vi "Modbus RT Driver DEBUG Simulate Data.vi"(8 "error in (no error)":errorcluster) -> (0 "error out":errorcluster, 1 "DEBUG RT-FIFOs Indexes":T2[](array[typedef]), 2 "DEBUG Modbus Items":T4[](array[typedef]), 5 "Input Specified Channel Ref List":T1[](array[typedef]) format="%.0x", 7 "Output Specified Channel Ref List":T1[](array[typedef]) format="%.0x")   [LabVIEW 2014, in "Modbus Engine.lvlib"]
uses:
  Modbus Engine.lvlib
  XML Deserializer/XML VIs/API/Controls/Modbus_Items.ctl
  XML Deserializer/XML VIs/API/Controls/Modbus_Item_Type.ctl
  Shared/FIFO Indexes.ctl
  <vilib>/NI Veristand/Custom Device API/Custom Device Channel Type.ctl
  <vilib>/NI Veristand/Custom Device API/Custom Device Item Ref.ctl
  <vilib>/NI Veristand/Custom Device API/Custom Device API.lvlib
  Shared/Modbus Shared.lvlib
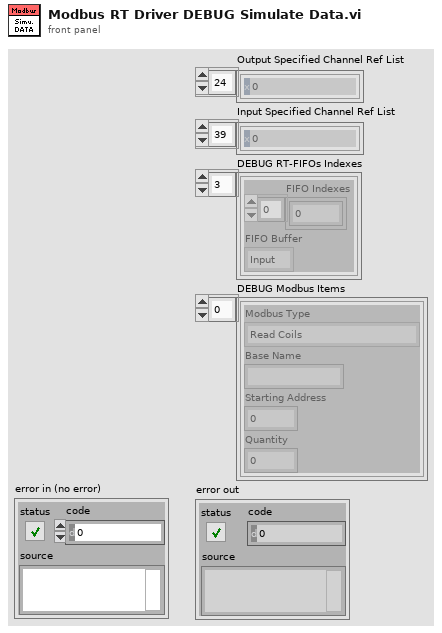
[diagram p1: front panel]
types:
  T1 = typedef "Custom Device API.lvlib/Custom Device Item Ref.ctl" = u64
  T2 = typedef "Modbus Shared.lvlib/FIFO Indexes.ctl" = cluster{"FIFO Indexes":i32[], "FIFO Buffer":T3}
  T3 = typedef "Custom Device API.lvlib/Custom Device Channel Type.ctl" = enum16{"Input", "Output"}
  T4 = typedef "Modbus Shared.lvlib/Modbus_Items.ctl" = cluster{"Modbus Type":T5, "Base Name":string, "Starting Address":u16, "Quantity":u16}
  T5 = typedef "Modbus Shared.lvlib/Modbus_Item_Type.ctl" = enum16{"Read Coils", "Read Discrete Inputs", "Read Holding Registers", "Read Input Registers", "Write Multiple Coils", "Write Multiple Holding Registers", "Write Single Coil", "Write Single Holding Register", "Write Multiple Discrete Inputs", "Write Multiple Input Registers"}
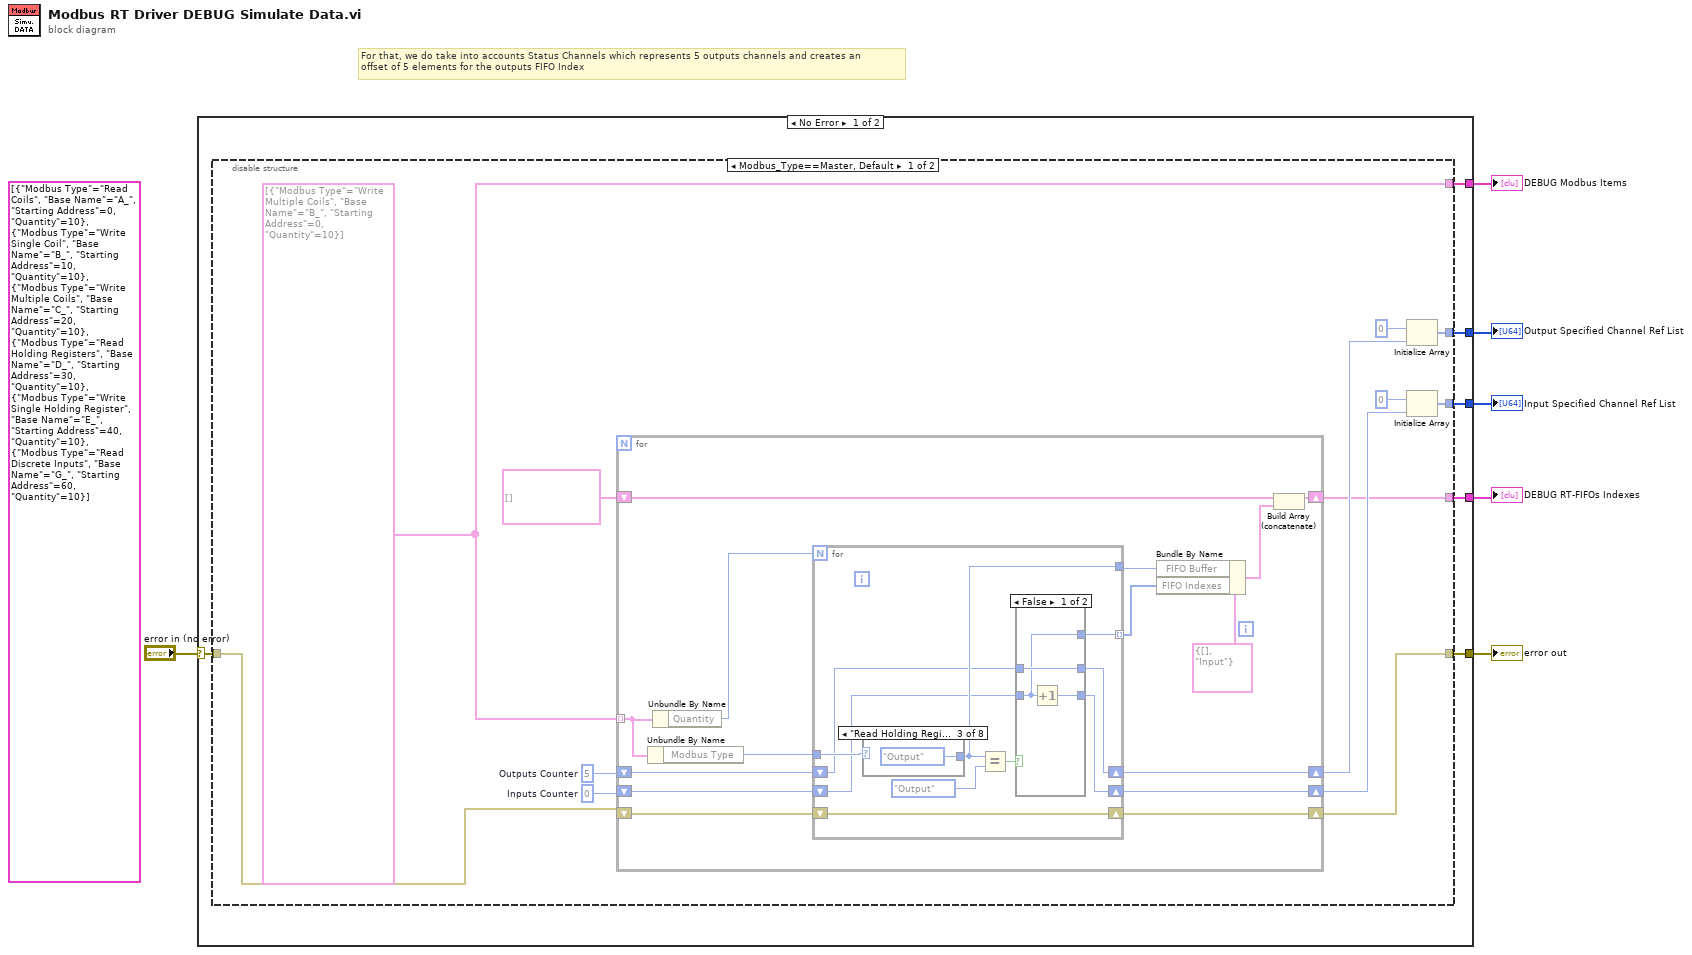
[diagram p0: block diagram]
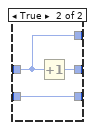
[diagram p2: hidden frame]
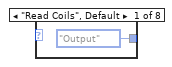
[diagram p3: hidden frame]
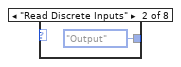
[diagram p4: hidden frame]
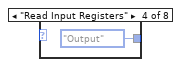
[diagram p5: hidden frame]
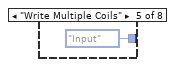
[diagram p6: hidden frame]
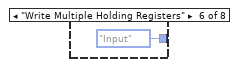
[diagram p7: hidden frame]
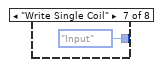
[diagram p8: hidden frame]
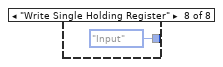
[diagram p9: hidden frame]
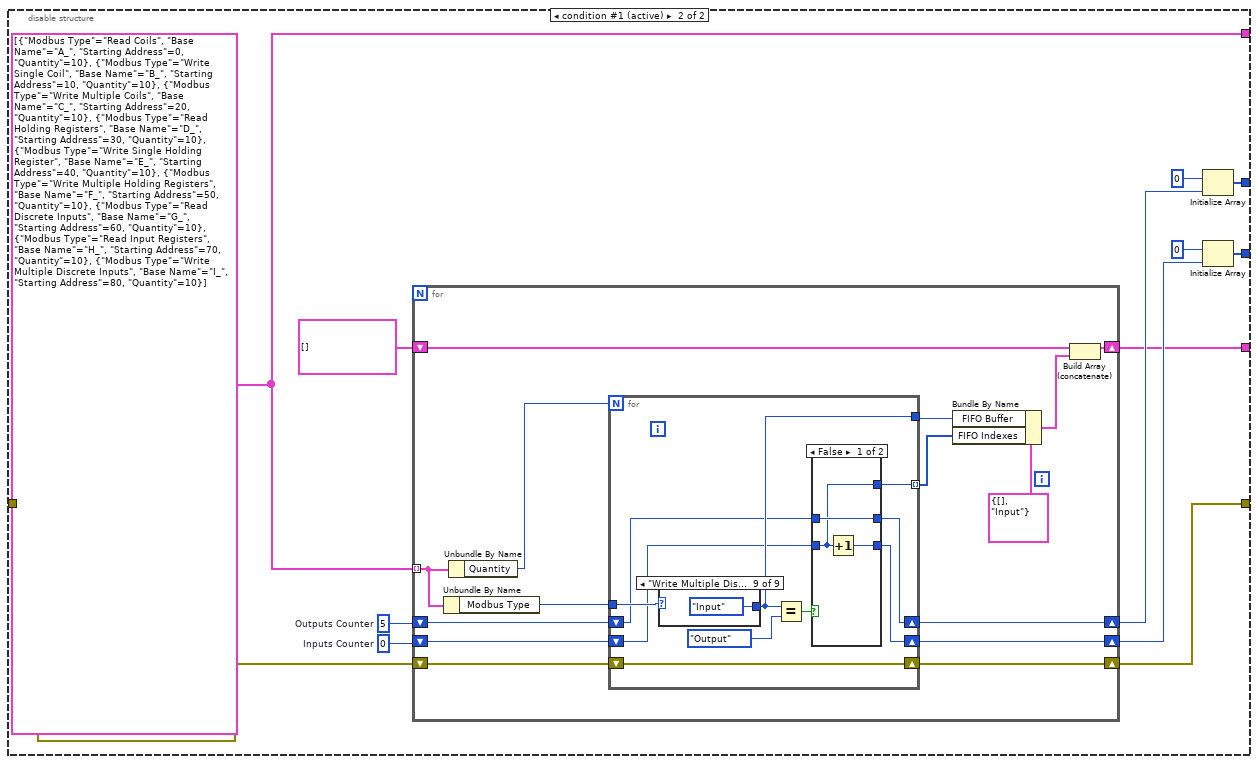
[diagram p10: hidden frame]
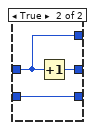
[diagram p11: hidden frame]
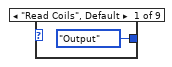
[diagram p12: hidden frame]
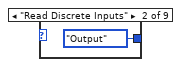
[diagram p13: hidden frame]
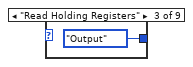
[diagram p14: hidden frame]
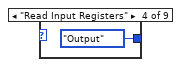
[diagram p15: hidden frame]
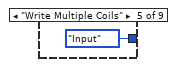
[diagram p16: hidden frame]
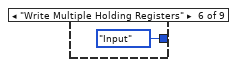
[diagram p17: hidden frame]
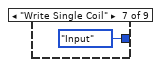
[diagram p18: hidden frame]
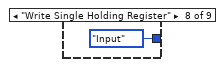
[diagram p19: hidden frame]
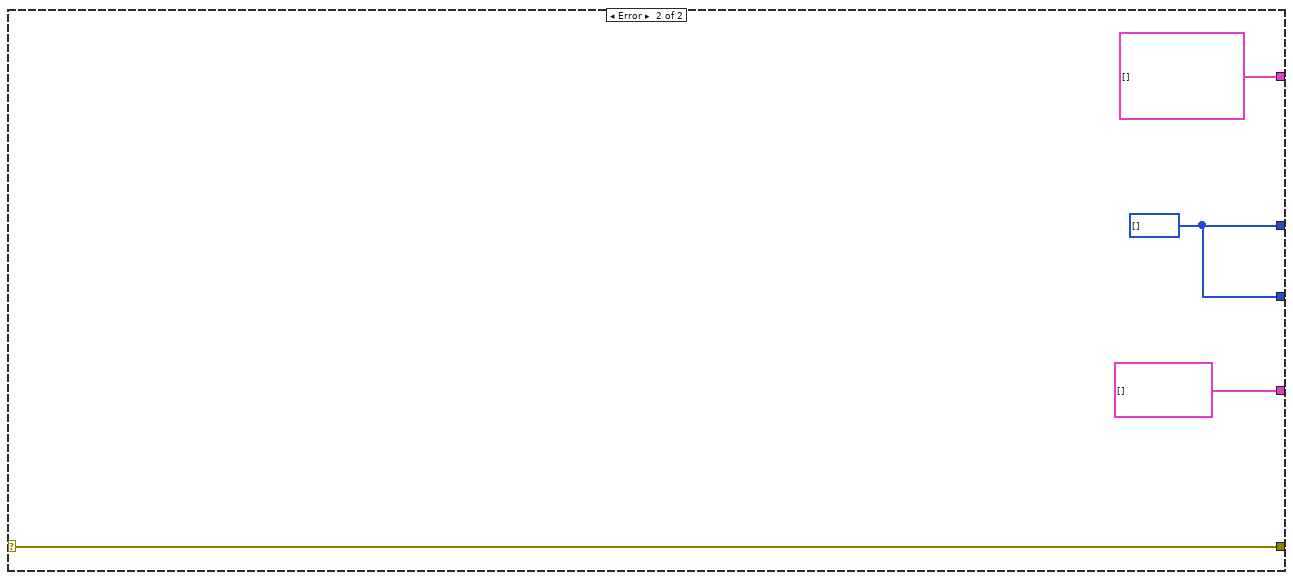
[diagram p20: hidden frame]
diagram:
  (unwired) T4[] [{"Modbus Type"=enum."Read Coils", "Base Name"="A_", "Starting Address"=0, "Quantity"=10}, {"Modbus Type"=enum."Write Single Coil", "Base Name"="B_", "Starting Address"=10, "Quantity"=10}, {"Modbus Type"=enum."Write Multiple Coils", "Base Name"="C_", "Starting Address"=20, "Quantity"=10}, {"Modbus Type"=enum."Read Holding Registers", "Base Name"="D_", "Starting Address"=30, "Quantity"=10}, {"Modbus Type"=enum."Write Single Holding Register", "Base Name"="E_", "Starting Address"=40, "Quantity"=10}, {"Modbus Type"=enum."Read Discrete Inputs", "Base Name"="G_", "Starting Address"=60, "Quantity"=10}] ("DEBUG Modbus Items")
  # "For that, we do take into accounts Status Channels which represents 5 outputs channels and creates an \noffset of 5 elements for the outputs FIFO Index"
  n1 = case shown="No Error" "error in (no error)" {
    selector: "error in (no error)" -> [w12 w121]
    tunnel: [w11 w121] -> w5
    tunnel: [w9 w120] -> w4
    tunnel: [w8 w120] -> w3
    tunnel: [w7 T2[] [] ("DEBUG RT-FIFOs Indexes")] -> w2
    tunnel: [w10 T4[] [] ("DEBUG Modbus Items")] -> w1
    frame No Error {
      n2 = disable-structure shown="Modbus_Type==Master, Default" {
        disable-tunnel: w12 -> [w21 w73]
        disable-tunnel: [w20 w72] -> w11
        disable-tunnel: [w19 w71] -> w10
        disable-tunnel: [w24 w76] -> w9
        disable-tunnel: [w22 w74] -> w8
        disable-tunnel: [w13 w65] -> w7
        frame condition #0 {
          w17 = 0  # Inputs Counter
          w18 = 5  # Outputs Counter
          w19 = T4[] [{"Modbus Type"=enum."Write Multiple Coils", "Base Name"="B_", "Starting Address"=0, "Quantity"=10}] ("DEBUG Modbus Items")
          n3 = for {
            shift-right: [w39] -> w20
            shift-left: w21 -> [w40]
            shift-right: [w27] -> w16
            shift-left: w18 -> [w30]
            shift-right: [w26] -> w15
            shift-left: w17 -> [w29]
            tunnel: w19 -> [w37] mode=indexing
            shift-right: [w31] -> w13
            shift-left: T2[] [] ("DEBUG RT-FIFOs Indexes") -> [w32]
            n4 = Unbundle By Name(w37) -> ("Modbus Type"=w38:T5)
            n5 = Unbundle By Name(w37) -> ("Quantity"=w36:u16)
            n6 = for {
              N: w36 -> [_]
              shift-right: [w49] -> w39
              shift-left: w40 -> [w49]
              tunnel: w38 -> [w50]
              tunnel: [w46] -> w34
              shift-right: [w45] -> w26
              shift-left: w29 -> [w42]
              shift-right: [w44] -> w27
              shift-left: w30 -> [w43]
              tunnel: [w41] -> w28 mode=indexing
              n7 = case shown="\"Read Holding Registers\"" w50 {
                tunnel: [Custom_Device_Channel_Type."Output" ("Type") Custom_Device_Channel_Type."Output" ("Type") Custom_Device_Channel_Type."Output" ("Type") Custom_Device_Channel_Type."Output" ("Type") Custom_Device_Channel_Type."Input" ("Type") Custom_Device_Channel_Type."Input" ("Type") Custom_Device_Channel_Type."Input" ("Type") Custom_Device_Channel_Type."Input" ("Type")] -> w46
                frame "Read Coils", Default {
                }
                frame "Read Discrete Inputs" {
                }
                frame "Read Holding Registers" {
                }
                frame "Read Input Registers" {
                }
                frame "Write Multiple Coils" {
                }
                frame "Write Multiple Holding Registers" {
                }
                frame "Write Single Coil" {
                }
                frame "Write Single Holding Register" {
                }
              }
              n8 = Equal?(x=w46, y=Custom_Device_Channel_Type."Output") -> (x = y?=w47:bool)
              n9 = case shown="False" w47 {
                tunnel: w43 -> [w53 w54]
                tunnel: w42 -> [w51 w55]
                tunnel: [w53 w56] -> w44
                tunnel: [w52 w55] -> w45
                tunnel: [w51 w54] -> w41
                frame False {
                  n10 = Increment(x=w51) -> (x+1=w52:i32)
                }
                frame True {
                  n11 = Increment(x=w54) -> (x+1=w56:i32)
                }
              }
            }
            n12 = Bundle By Name(cluster=T2 {"FIFO Indexes"=[], "FIFO Buffer"=enum."Input"} ("Cluster"), "FIFO Buffer"=w34, "FIFO Indexes"=w28) -> (w33:T2)
            n13 = Build Array (concatenate)(w32, w33) -> (w31:T2[])
          }
          n14 = Initialize Array(T1 0 ("Device Item Ref"), w16) -> (w24:T1[])
          n15 = Initialize Array(T1 0 ("Device Item Ref"), w15) -> (w22:T1[])
        }
        frame condition #1 (active) {
          w69 = 0  # Inputs Counter
          w70 = 5  # Outputs Counter
          w71 = T4[] [{"Modbus Type"=enum."Read Coils", "Base Name"="A_", "Starting Address"=0, "Quantity"=10}, {"Modbus Type"=enum."Write Single Coil", "Base Name"="B_", "Starting Address"=10, "Quantity"=10}, {"Modbus Type"=enum."Write Multiple Coils", "Base Name"="C_", "Starting Address"=20, "Quantity"=10}, {"Modbus Type"=enum."Read Holding Registers", "Base Name"="D_", "Starting Address"=30, "Quantity"=10}, {"Modbus Type"=enum."Write Single Holding Register", "Base Name"="E_", "Starting Address"=40, "Quantity"=10}, {"Modbus Type"=enum."Write Multiple Holding Registers", "Base Name"="F_", "Starting Address"=50, "Quantity"=10}, {"Modbus Type"=enum."Read Discrete Inputs", "Base Name"="G_", "Starting Address"=60, "Quantity"=10}, {"Modbus Type"=enum."Read Input Registers", "Base Name"="H_", "Starting Address"=70, "Quantity"=10}, {"Modbus Type"=enum."Write Multiple Discrete Inputs", "Base Name"="I_", "Starting Address"=80, "Quantity"=10}] ("DEBUG Modbus Items")
          n16 = for {
            shift-right: [w91] -> w72
            shift-left: w73 -> [w92]
            shift-right: [w79] -> w68
            shift-left: w70 -> [w82]
            shift-right: [w78] -> w67
            shift-left: w69 -> [w81]
            tunnel: w71 -> [w89] mode=indexing
            shift-right: [w83] -> w65
            shift-left: T2[] [] ("DEBUG RT-FIFOs Indexes") -> [w84]
            n17 = Unbundle By Name(w89) -> ("Modbus Type"=w90:T5)
            n18 = Unbundle By Name(w89) -> ("Quantity"=w88:u16)
            n19 = for {
              N: w88 -> [_]
              shift-right: [w101] -> w91
              shift-left: w92 -> [w101]
              tunnel: w90 -> [w102]
              tunnel: [w98] -> w86
              shift-right: [w97] -> w78
              shift-left: w81 -> [w94]
              shift-right: [w96] -> w79
              shift-left: w82 -> [w95]
              tunnel: [w93] -> w80 mode=indexing
              n20 = case shown="\"Write Multiple Discrete Inputs\"" w102 {
                tunnel: [Custom_Device_Channel_Type."Output" ("Type") Custom_Device_Channel_Type."Output" ("Type") Custom_Device_Channel_Type."Output" ("Type") Custom_Device_Channel_Type."Output" ("Type") Custom_Device_Channel_Type."Input" ("Type") Custom_Device_Channel_Type."Input" ("Type") Custom_Device_Channel_Type."Input" ("Type") Custom_Device_Channel_Type."Input" ("Type") Custom_Device_Channel_Type."Input" ("Type")] -> w98
                frame "Read Coils", Default {
                }
                frame "Read Discrete Inputs" {
                }
                frame "Read Holding Registers" {
                }
                frame "Read Input Registers" {
                }
                frame "Write Multiple Coils" {
                }
                frame "Write Multiple Holding Registers" {
                }
                frame "Write Single Coil" {
                }
                frame "Write Single Holding Register" {
                }
                frame "Write Multiple Discrete Inputs" {
                }
              }
              n21 = Equal?(x=w98, y=Custom_Device_Channel_Type."Output") -> (x = y?=w99:bool)
              n22 = case shown="False" w99 {
                tunnel: w95 -> [w105 w106]
                tunnel: w94 -> [w103 w107]
                tunnel: [w105 w108] -> w96
                tunnel: [w104 w107] -> w97
                tunnel: [w103 w106] -> w93
                frame False {
                  n23 = Increment(x=w103) -> (x+1=w104:i32)
                }
                frame True {
                  n24 = Increment(x=w106) -> (x+1=w108:i32)
                }
              }
            }
            n25 = Bundle By Name(cluster=T2 {"FIFO Indexes"=[], "FIFO Buffer"=enum."Input"} ("Cluster"), "FIFO Buffer"=w86, "FIFO Indexes"=w80) -> (w85:T2)
            n26 = Build Array (concatenate)(w84, w85) -> (w83:T2[])
          }
          n27 = Initialize Array(T1 0 ("Device Item Ref"), w68) -> (w76:T1[])
          n28 = Initialize Array(T1 0 ("Device Item Ref"), w67) -> (w74:T1[])
        }
      }
    }
    frame Error {
      w120 = T1[] [] ("Output Specified Channel Ref List")
    }
  }
  "DEBUG Modbus Items" <- w1
  "DEBUG RT-FIFOs Indexes" <- w2
  "Output Specified Channel Ref List" <- w4
  "Input Specified Channel Ref List" <- w3
  "error out" <- w5
